vi "Write Teller.vi"(10 "Teller":refnum<class "Teller.lvclass">, 11 "Stopped Msg in":refnum<class "--Stopped Msg.lvclass">) -> (3 "Stopped Msg out":refnum<class "--Stopped Msg.lvclass">)   [LabVIEW 2025, in "jettl.lvlib" / "Stopped jettl Msg.lvlib" / "--Stopped Msg.lvclass"]
uses:
  --Stopped Msg.lvclass
  Teller/Teller.lvclass
  --Stopped Msg.lvclass/--Stopped Msg.ctl
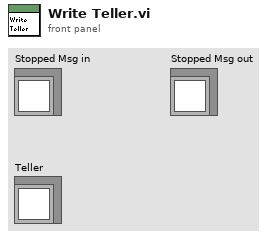
[diagram p1: front panel]
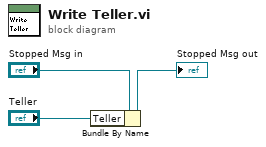
[diagram p0: block diagram]
diagram:
  n1 = Bundle By Name(cluster="Stopped Msg in", "Teller"="Teller") -> (→"Stopped Msg out":refnum<class "--Stopped Msg.lvclass">)
